vi "Avg Temps Flows Labels Data.vi"() -> (0 "FuelData":bool, 1 "AvgFuelsLabels":T1(array[cluster]), 2 "TempData":bool, 3 "AvgTempsLabels":T1(array[cluster]))   [LabVIEW 2017]
panel:
  in  "AvgTempLabels":T2
  in  "array":variant[](array[variant])
  in  "AvgFuelLabels":T2
  in  "array 2":variant[](array[variant])
  in  "Avg fuel":T3
  in  "output cluster":T3
  in  "dummy fuel array":dbl[][][](array[numeric])
  in  "Dummy Temp array":dbl[][][](array[numeric])
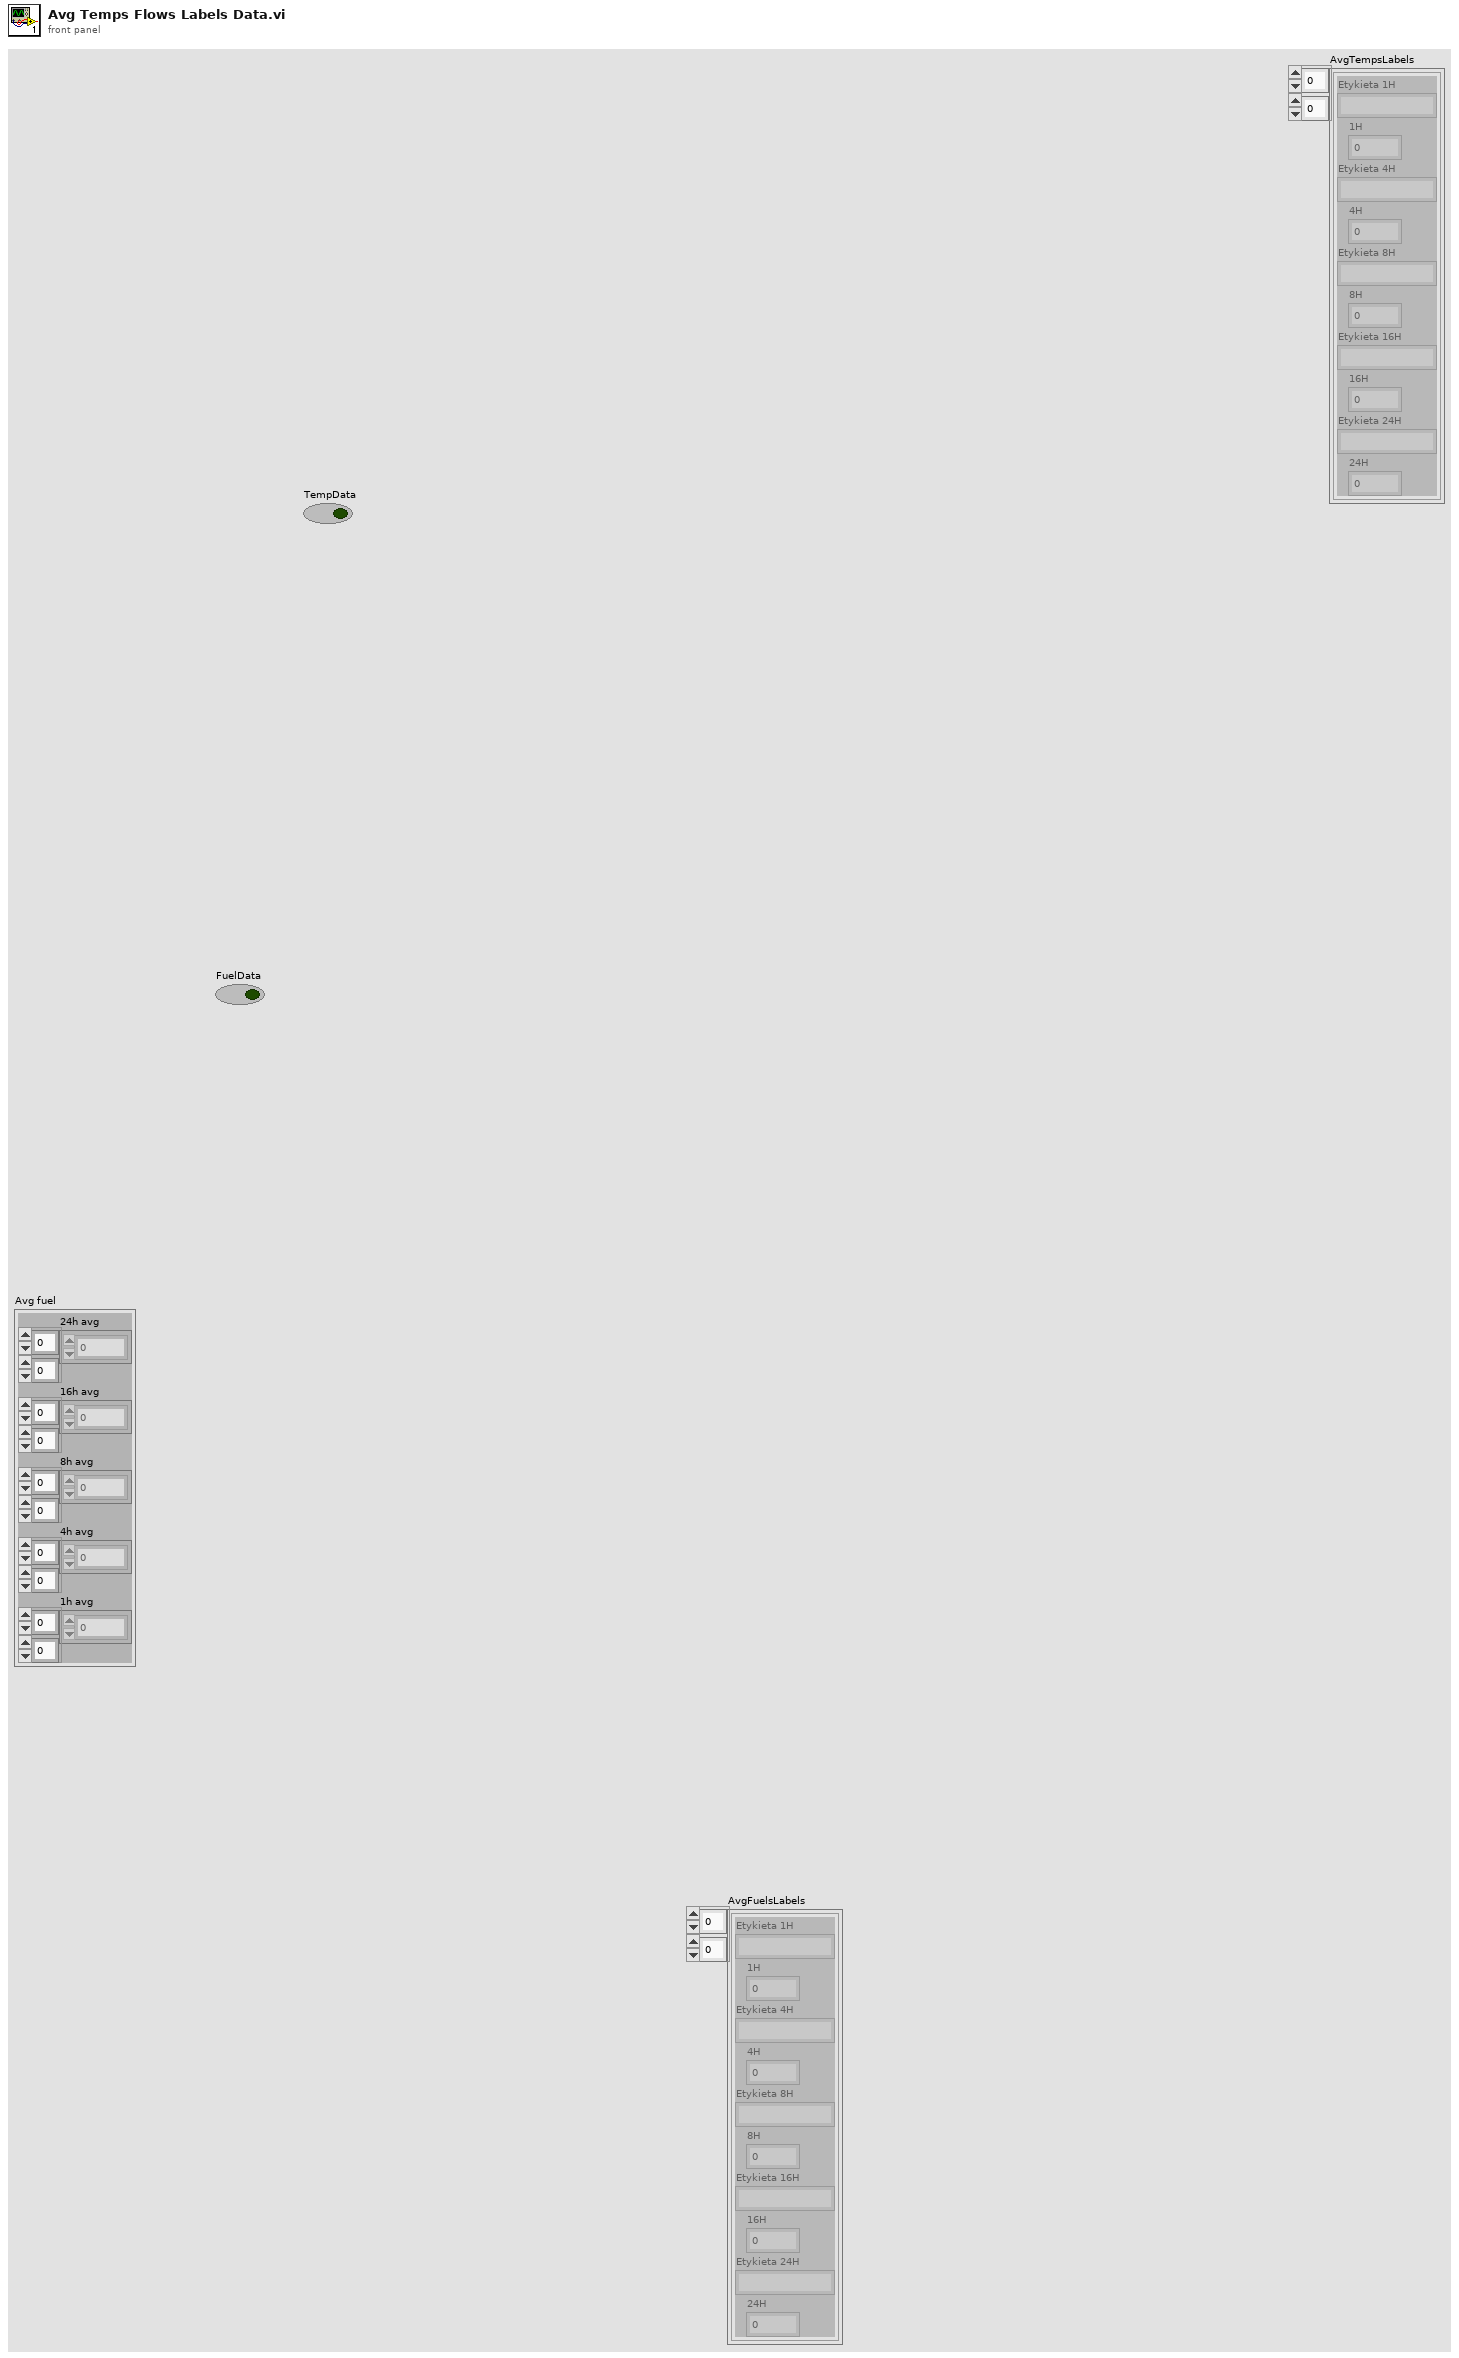
[diagram p1: front panel]
types:
  T1 = cluster{"Etykieta 1H":string, "1H":dbl, "Etykieta 4H":string, "4H":dbl, "Etykieta 8H":string, "8H":dbl, "Etykieta 16H":string, "16H":dbl, "Etykieta 24H":string, "24H":dbl}[][]
  T2 = cluster{"Etykieta 1H":string, "1H":dbl, "Etykieta 4H":string, "4H":dbl, "Etykieta 8H":string, "8H":dbl, "Etykieta 16H":string, "16H":dbl, "Etykieta 24H":string, "24H":dbl}
  T3 = cluster{"24h avg":dbl[][], "16h avg":dbl[][], "8h avg":dbl[][], "4h avg":dbl[][], "1h avg":dbl[][]}
  T4 = cluster{"Termometr 1":string, "Termometr 2":string, "Termometr 3":string, "Termometr 4":string, "Termometr 5":string, "Termometr 6":string, "Termometr 7":string, "Termometr 8":string, "Termometr 9":string, "Termometr 10":string}
  T5 = cluster{"Paliwo 1":string, "Paliwo 2":string, "Paliwo 3":string, "Paliwo 4":string, "Paliwo 5":string, "Paliwo 6":string}
  T6 = cluster{"array[0]":variant, "array[1]":variant, "array[2]":variant, "array[3]":variant, "array[4]":variant, "array[5]":variant, "array[6]":variant, "array[7]":variant, "array[8]":variant, "array[9]":variant}
  T7 = cluster{"array 2[0]":variant, "array 2[1]":variant, "array 2[2]":variant, "array 2[3]":variant, "array 2[4]":variant, "array 2[5]":variant, "array 2[6]":variant, "array 2[7]":variant, "array 2[8]":variant, "array 2[9]":variant}
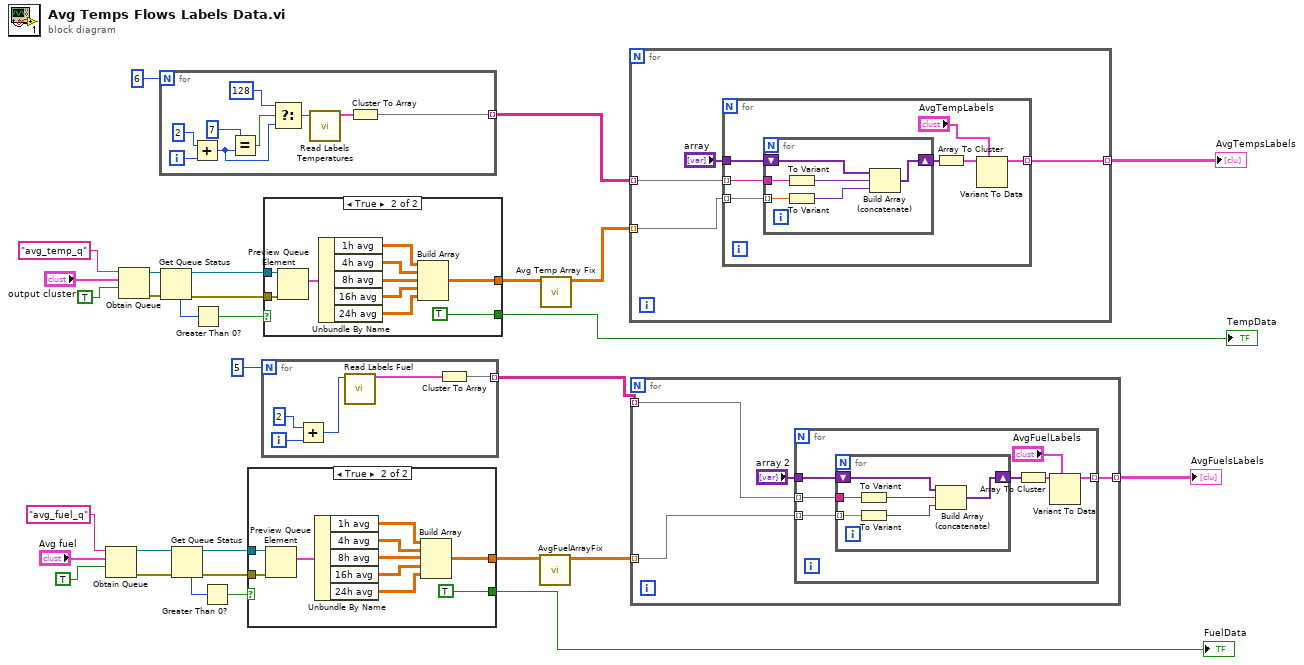
[diagram p0: block diagram]
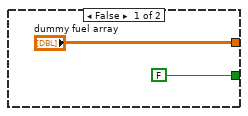
[diagram p2: hidden frame]
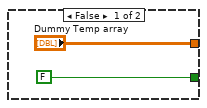
[diagram p3: hidden frame]
diagram:
  n1 = Obtain Queue(name (unnamed)="avg_fuel_q", element data type="Avg fuel", create if not found? (T)=TRUE) -> (queue out=w23:refnum<queue>, error out=w24:errorcluster)  [unwired: 2 in, 1 out]
  n2 = Obtain Queue(name (unnamed)="avg_temp_q", element data type="output cluster", create if not found? (T)=TRUE) -> (queue out=w14:refnum<queue>, error out=w13:errorcluster)  [unwired: 2 in, 1 out]
  n3 = for {
    N: 6 -> [_]
    tunnel: [w31] -> w30 mode=indexing
    i -> [w39]
    n4 = Add(x=2, y=w39) -> (x+y=w34:i32)
    n5 = Equal?(x=7, y=w34) -> (x = y?=w35:bool)
    n6 = Select(t=128, s=w35, f=w34) -> (s? t:f=w37:i32)
    n7 = call "Read Labels Temperatures.vi"("Slave ID"=w37) -> ("Etykiety T1-10"=w32:T4)  [unwired: 10 in]
    n8 = Cluster To Array(cluster=w32) -> (array=w31:string[])
  }
  n9 = Get Queue Status(queue=w14, error in (no error)=w13) -> (queue out=w9:refnum<queue>, error out=w8:errorcluster, # elements in queue=w7:i32)  [unwired: 1 in, 5 out]
  n10 = Get Queue Status(queue=w23, error in (no error)=w24) -> (queue out=w21:refnum<queue>, error out=w20:errorcluster, # elements in queue=w18:i32)  [unwired: 1 in, 5 out]
  n11 = Greater Than 0?(x=w7) -> (x > 0?=w10:bool)
  n12 = Greater Than 0?(x=w18) -> (x > 0?=w19:bool)
  n13 = case shown="True" w19 {
    tunnel: w21 -> [_ w51]
    tunnel: w20 -> [_ w50]
    tunnel: [FALSE TRUE] -> w25
    tunnel: ["dummy fuel array" w48] -> w6
    frame False {
    }
    frame True {
      n14 = Preview Queue Element(queue=w51, error in (no error)=w50) -> (element=w47:T3)  [unwired: 1 in, 3 out]
      n15 = Unbundle By Name(w47) -> ("1h avg"=w42:dbl[][], "4h avg"=w45:dbl[][], "8h avg"=w46:dbl[][], "16h avg"=w43:dbl[][], "24h avg"=w44:dbl[][])
      n16 = Build Array(w42, w45, w46, w43, w44) -> (w48:dbl[][][])
    }
  }
  "FuelData" <- w25
  n17 = for {
    N: 5 -> [_]
    tunnel: [w53] -> w4 mode=indexing
    i -> [w56]
    n18 = Add(x=2, y=w56) -> (x+y=w54:i32)
    n19 = call "Read Labels Fuel.vi"("Slave ID"=w54) -> ("Etykiety P1-6"=w52:T5)  [unwired: 10 in]
    n20 = Cluster To Array(cluster=w52) -> (array=w53:string[])
  }
  n21 = case shown="True" w10 {
    tunnel: w8 -> [_ w67]
    tunnel: w9 -> [_ w68]
    tunnel: [FALSE TRUE] -> w15
    tunnel: ["Dummy Temp array" w59] -> w2
    frame False {
    }
    frame True {
      n22 = Preview Queue Element(queue=w68, error in (no error)=w67) -> (element=w65:T3)  [unwired: 1 in, 3 out]
      n23 = Unbundle By Name(w65) -> ("1h avg"=w60:dbl[][], "4h avg"=w64:dbl[][], "8h avg"=w63:dbl[][], "16h avg"=w61:dbl[][], "24h avg"=w62:dbl[][])
      n24 = Build Array(w60, w64, w63, w61, w62) -> (w59:dbl[][][])
    }
  }
  "TempData" <- w15
  n25 = call "AvgFuelArrayFix.vi"("AvgFuelArrayin"=w6) -> ("AvgFuelArrayout"=w5:dbl[][][])  [unwired: 10 in]
  n26 = call "Avg Temp Array Fix.vi"("Input Array"=w2) -> ("Output Array"=w1:dbl[][][])  [unwired: 10 in]
  n27 = for {
    tunnel: w30 -> [w72] mode=indexing
    tunnel: [w70] -> w29 mode=indexing
    tunnel: w1 -> [w69] mode=indexing
    n28 = for {
      tunnel: w69 -> [w78] mode=indexing
      tunnel: w72 -> [w79] mode=indexing
      tunnel: "array" -> [w77]
      tunnel: [w74] -> w70 mode=indexing
      n29 = for {
        tunnel: w79 -> [w84]
        tunnel: w78 -> [w85] mode=indexing
        shift-right: [w82] -> w76
        shift-left: w77 -> [w83]
        n30 = To Variant(anything=w84) -> (Variant=w81:variant)
        n31 = To Variant(anything=w85) -> (Variant=w80:variant)
        n32 = Build Array (concatenate)(w83, w81, w80) -> (w82:variant[])
      }
      n33 = Array To Cluster(array=w76) -> (cluster=w75:T6)
      n34 = Variant To Data(type="AvgTempLabels", Variant=w75) -> (data=w74:T2)  [unwired: 1 in, 1 out]
    }
  }
  "AvgTempsLabels" <- w29
  n35 = for {
    tunnel: w4 -> [w88] mode=indexing
    tunnel: [w87] -> w3 mode=indexing
    tunnel: w5 -> [w86] mode=indexing
    n36 = for {
      tunnel: w86 -> [w95] mode=indexing
      tunnel: w88 -> [w96] mode=indexing
      tunnel: "array 2" -> [w94]
      tunnel: [w91] -> w87 mode=indexing
      n37 = for {
        tunnel: w96 -> [w101]
        tunnel: w95 -> [w102] mode=indexing
        shift-right: [w97] -> w90
        shift-left: w94 -> [w100]
        n38 = To Variant(anything=w101) -> (Variant=w99:variant)
        n39 = To Variant(anything=w102) -> (Variant=w98:variant)
        n40 = Build Array (concatenate)(w100, w99, w98) -> (w97:variant[])
      }
      n41 = Array To Cluster(array=w90) -> (cluster=w93:T7)
      n42 = Variant To Data(type="AvgFuelLabels", Variant=w93) -> (data=w91:T2)  [unwired: 1 in, 1 out]
    }
  }
  "AvgFuelsLabels" <- w3
